vi "Conv_Rotations_Degrees.vi"(10 "Rotations":dbl) -> (2 "Degrees":dbl)   [LabVIEW 2019, in "Trajectory_Library.lvlib"]
doc: "Convert Rotations to Degrees"
uses:
  Trajectory_Library.lvlib
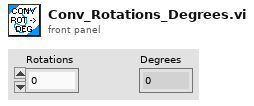
[diagram p1: front panel]
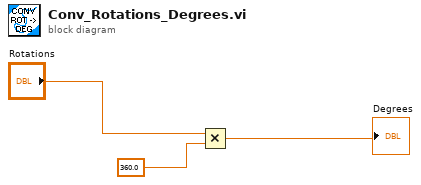
[diagram p0: block diagram]
diagram:
  n1 = Multiply(x="Rotations", y=360.0) -> (x*y=→"Degrees":dbl)
